vi "Cross Array Main.vi"() -> ()   [LabVIEW 2014]
uses:
  Slicer/LVslicer/Slice/TypeDefs/PowerSpeed.ctl
  Slicer/LVslicer/Slice/TypeDefs/PathSupreme.ctl
  Slicer/LVslicer/Slice/OverhangParam/PSup2SCAN/Sub/VelocityProfile.ctl
  Slicer/LVslicer/Slice/OverhangParam/PSup2SCAN/Sub/PathCut.ctl
  Slicer/LVslicer/Slice/OverhangParam/PSup2SCAN/Sub/Segment.ctl
  Slicer_11-28/LVslicer/Slice/TypeDefs/Point3D.ctl
  <vilib>/picture/3D Picture Control/Object/Create Object (name).vi
  <vilib>/picture/3D Picture Control/NI_3D Picture Control.lvlib
panel:
  in  "Layer Thickness":dbl
  in  "Path":path
  out "PathSupreams":T1[](array[typedef])
  in  "save":bool
  in  "Spacing":dbl
  in  "Plate \nDiameter":dbl
  out "Stoped":bool
  in  "HighPower":dbl=500.0
  in  "Display":T5={"Mode"=enum."Inherit Value", "PointSize"=1.0, "LineWidth"=1.0}
  out "3D Picture":refnum<vi>(3d-picture)
  out "PathSupreme":T1
  in  "stop":bool
  in  "Create Array":bool
  in  "Create Cross":bool
  in  "Beam Width":dbl
  in  "Cross X dimension\n(cross is square)":dbl
  in  "HatchPower":T6={"Power"=300.0, "Mark Speed"=400.0, "Jump Speed"=1000.0}
  # "* All dimensions are in mm's"
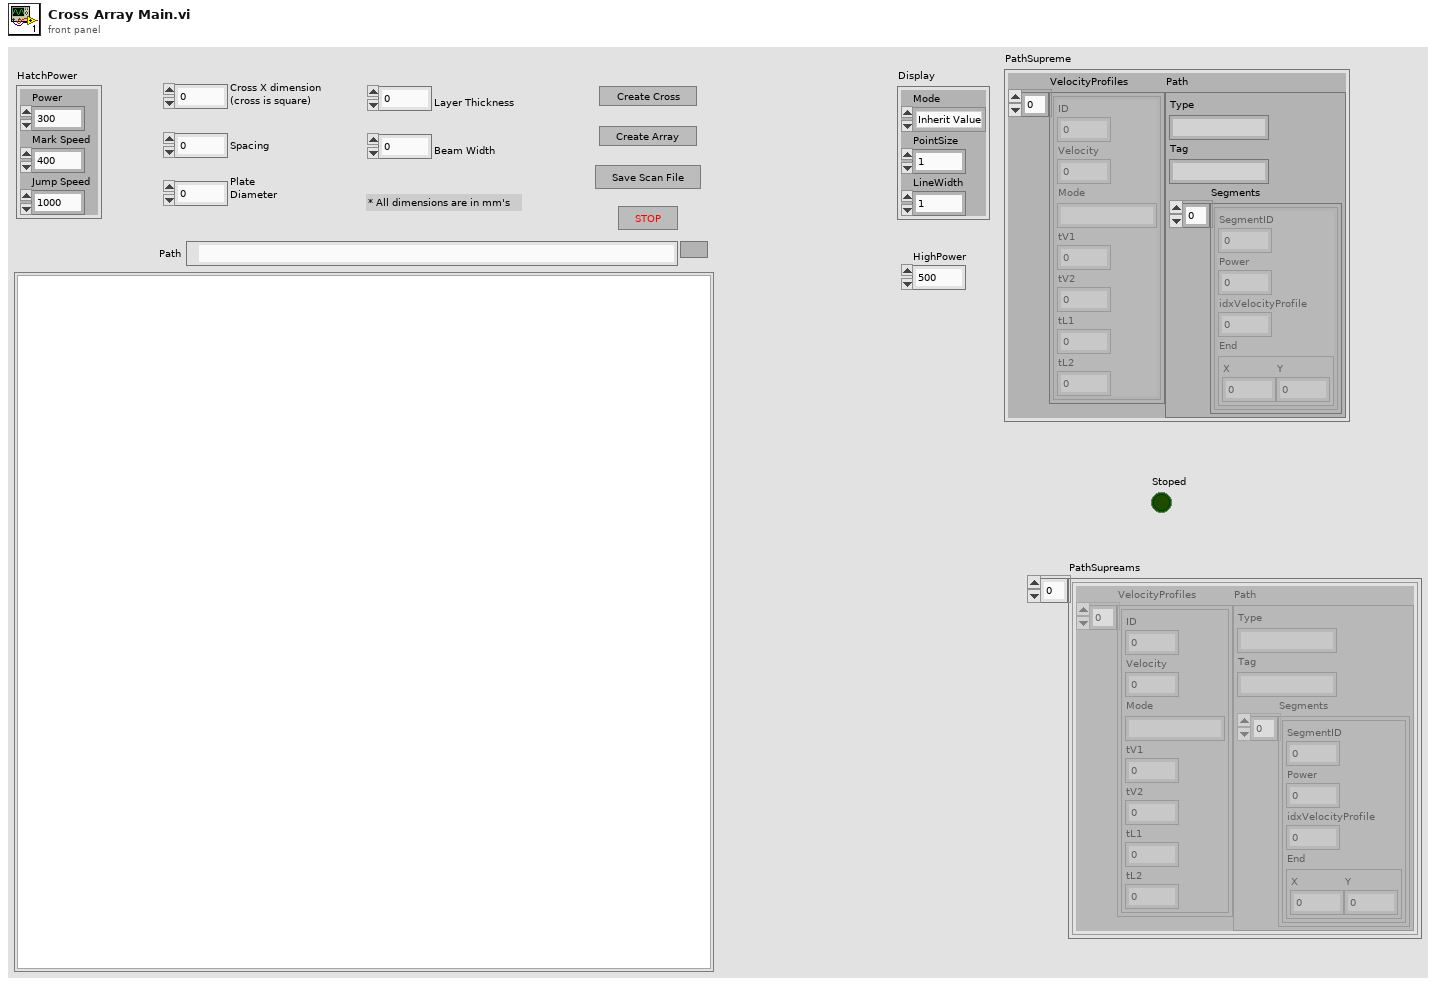
[diagram p1: front panel]
types:
  T1 = typedef "PathSupreme.ctl" = cluster{"VelocityProfiles":T2[], "Path":T3}
  T2 = typedef "VelocityProfile.ctl" = cluster{"ID":u32, "Velocity":dbl, "Mode":string, "tV1":u32, "tV2":u32, "tL1":u32, "tL2":u32}
  T3 = typedef "PathCut.ctl" = cluster{"Type":string, "Tag":string, "Segments":T4[]}
  T4 = typedef "Segment.ctl" = cluster{"SegmentID":u16, "Power":sgl, "idxVelocityProfile":u16, "End":cluster{"X":sgl, "Y":sgl}}
  T5 = cluster{"Mode":enum16{"Inherit Value", "Points", "Wireframe", "Polygons"}, "PointSize":sgl, "LineWidth":sgl}
  T6 = typedef "PowerSpeed.ctl" = cluster{"Power":dbl, "Mark Speed":dbl, "Jump Speed":dbl}
  T7 = typedef "Point3D.ctl" = cluster{"X":sgl, "Y":sgl, "Z":sgl}
  T8 = cluster{"Lines":cluster{"P0":T7, "P1":T7}[], "Colors":u32[]}
  T9 = enum16{"Idle", "Wait", "Create Cross", "Create Array", "Stop"}
  T10 = typedef "Point2DwSlope.ctl" = cluster{"X":sgl, "Y":sgl, "Slope":dbl}
  T11 = cluster{"VertexArray":T10[], "OnOffAr":enum16{"On", "Off"}[]}
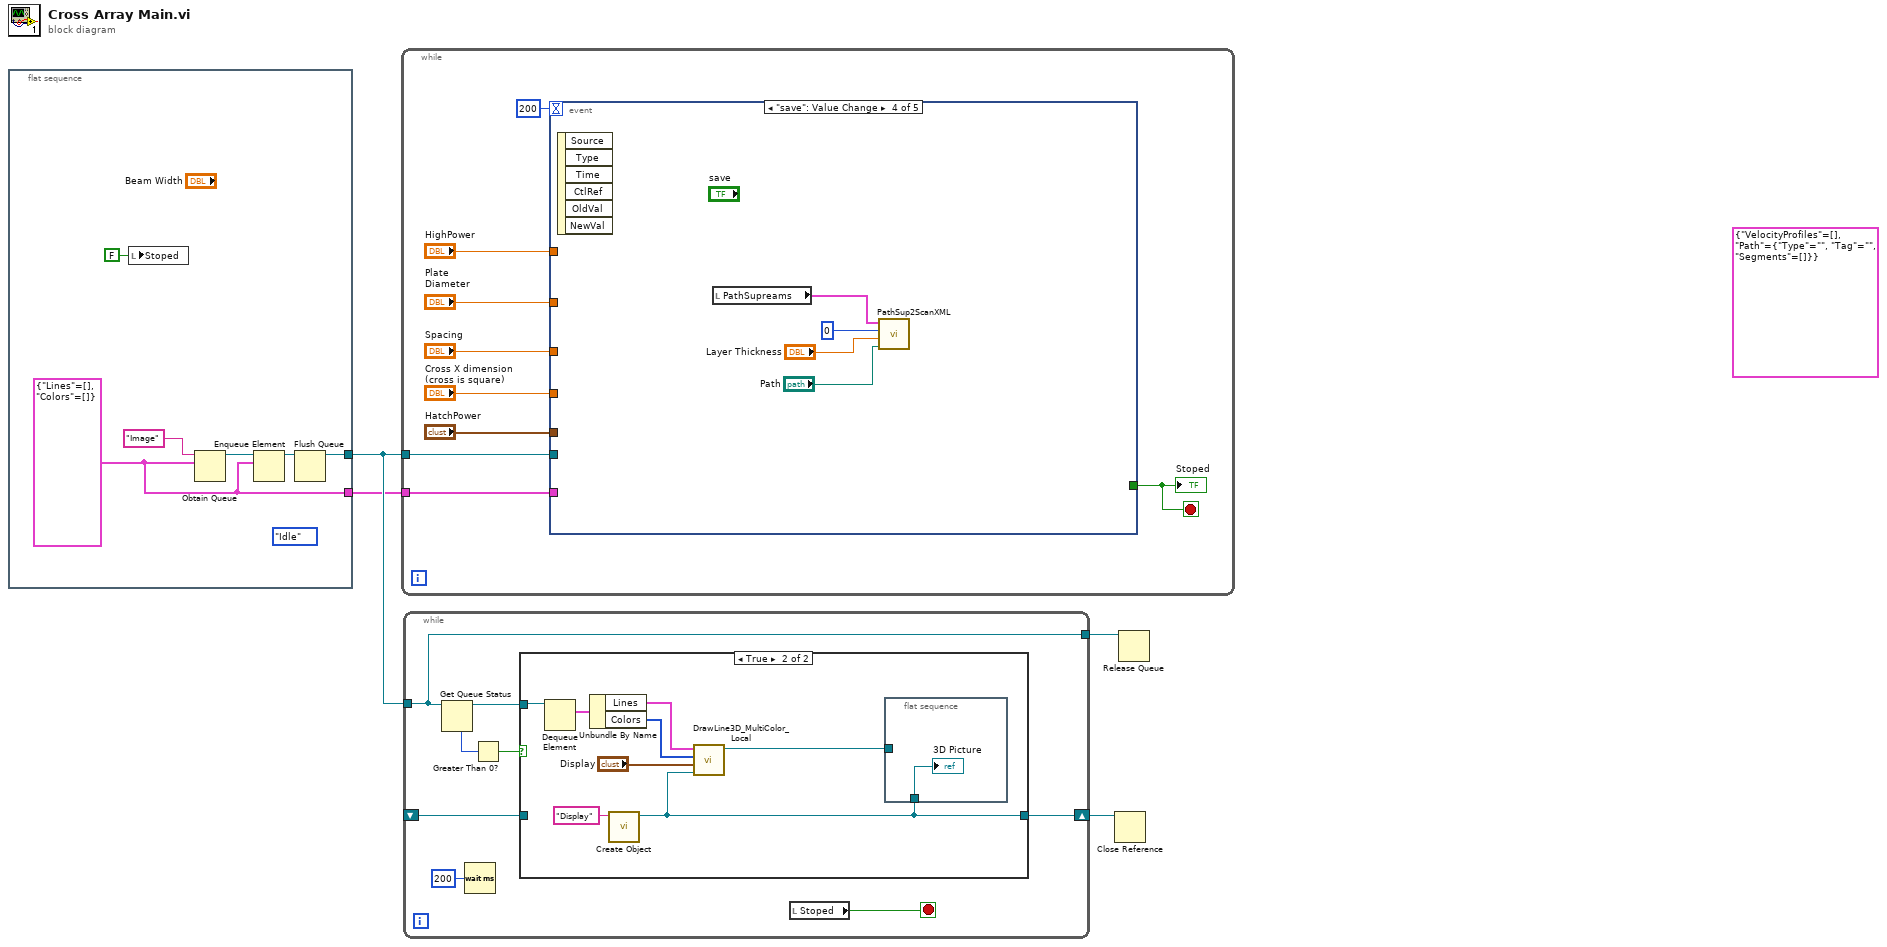
[diagram p0: block diagram]
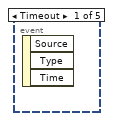
[diagram p2: hidden frame]
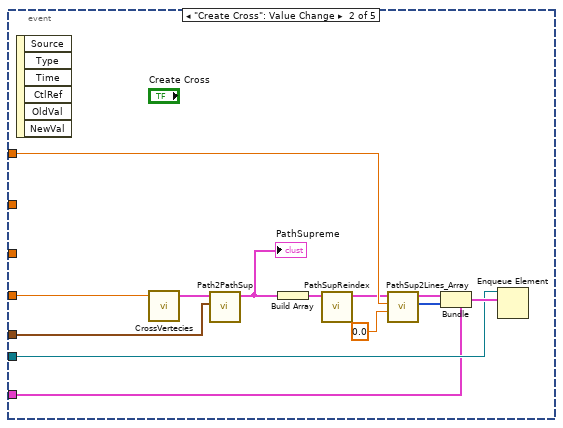
[diagram p3: hidden frame]
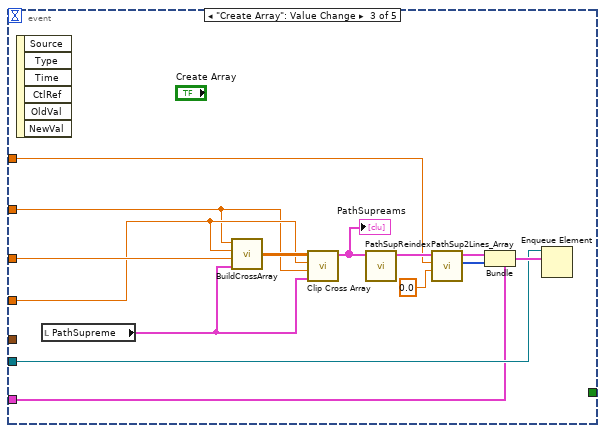
[diagram p4: hidden frame]
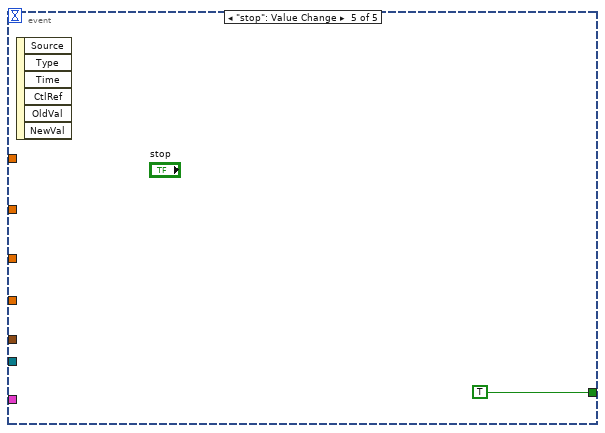
[diagram p5: hidden frame]
diagram:
  (unwired) T1 {"VelocityProfiles"=[], "Path"={"Type"="", "Tag"="", "Segments"=[]}} ("PathSupreme")
  n1 = flat-sequence {
    tunnel: [w7] -> w4
    tunnel: [w6] -> w3
    frame #0 {
      w6 = T8 {"Lines"=[], "Colors"=[]} ("output cluster")
      (unwired) T9."Idle" ("Action")
      n2 = local write "Stoped"(FALSE ("Stoped")) -> ()
      n3 = Obtain Queue(name (unnamed)="Image", element data type=w6) -> (queue out=w9:refnum<queue>)  [unwired: 3 in, 2 out]
      n4 = Enqueue Element(queue=w9, element=w6) -> (queue out=w8:refnum<queue>)  [unwired: 2 in, 2 out]
      n5 = Flush Queue(queue=w8) -> (queue out=w7:refnum<queue>)  [unwired: 1 in, 2 out]
    }
  }
  n6 = while {
    tunnel: w4 -> [w13]
    tunnel: w3 -> [w19]
    stop <- w18 stop-if-true
    n7 = event shown="[3] \"save\": Value Change" {
      selector: _ -> [_ _ _ _ _]
      dyn-events: _ -> [_ _ _ _ _]
      timeout: 200 -> [_ _ _ _ _]
      tunnel: "HighPower" -> [_ w31 w40 _ _]
      tunnel: w13 -> [_ w24 w39 _ _]
      tunnel: w19 -> [_ w23 w38 _ _]
      tunnel: [_ _ _ _ TRUE] -> w18
      tunnel: "Cross X dimension\n(cross is square)" -> [_ w21 w36 _ _]
      tunnel: "HatchPower" -> [_ w20 _ _ _]
      tunnel: "Plate \nDiameter" -> [_ _ w35 _ _]
      tunnel: "Spacing" -> [_ _ w46 _ _]
      event Timeout {
        n8 = event-data() -> ()  [unwired: 1 in, 3 out]
      }
      event "Create Cross": Value Change {
        n9 = event-data() -> ()  [unwired: 1 in, 6 out]
        n10 = call "CrossVertecies.vi"("Cross X dimension\n(cross is square)"=w21) -> ("Combined"=w32:T11)  [unwired: 4 in]
        n11 = call "Path2PathSup.vi"("PowerSpeed"=w20, "Combined"=w32) -> ("PathSupreme"=w22:T1)  [unwired: 9 in]
        "PathSupreme" <- w22
        n12 = Build Array(w22) -> (w28:T1[])
        n13 = call "PathSupReindex.vi"("PathSupremes"=w28) -> ("PathSupOut"=w29:T1[])  [unwired: 10 in]
        n14 = call "PathSup2Lines_Array.vi"("Z"=0.0, "HighPower"=w31, "PathSupIn"=w29) -> ("Colors"=w26:u32[], "Lines"=w27:cluster{"P0":T7, "P1":T7}[])  [unwired: 7 in]
        n15 = Bundle(cluster=w23, "Lines"=w27, "Colors"=w26) -> (w25:T8)
        n16 = Enqueue Element(queue=w24, element=w25) -> ()  [unwired: 2 in, 3 out]
      }
      event "Create Array": Value Change {
        n17 = event-data() -> ()  [unwired: 1 in, 6 out]
        n18 = local read "PathSupreme"() -> (w34:T1)
        n19 = call "BuildCrossArray.vi"("Plate \nDiameter (mm)"=w35, "Cross X dimension\n(cross is square)"=w36, "Desired\nSpacing(mm)"=w46, "PathSupreme"=w34) -> ("Array 2"=w37:dbl[][])  [unwired: 3 in, 1 out]
        n20 = call "Clip Cross Array.vi"("PathSupreme"=w34, "Plate \nDiameter (mm)"=w35, "Cross X dimension\n(cross is square)"=w36, "Origion Array"=w37) -> ("PathSupreams"=w33:T1[])  [unwired: 4 in]
        "PathSupreams" <- w33
        n21 = call "PathSupReindex.vi"("PathSupremes"=w33) -> ("PathSupOut"=w44:T1[])  [unwired: 10 in]
        n22 = call "PathSup2Lines_Array.vi"("Z"=0.0, "HighPower"=w40, "PathSupIn"=w44) -> ("Colors"=w42:u32[], "Lines"=w43:cluster{"P0":T7, "P1":T7}[])  [unwired: 7 in]
        n23 = Bundle(cluster=w38, "Lines"=w43, "Colors"=w42) -> (w41:T8)
        n24 = Enqueue Element(queue=w39, element=w41) -> ()  [unwired: 2 in, 3 out]
      }
      event "save": Value Change {
        n25 = event-data() -> ()  [unwired: 1 in, 6 out]
        n26 = local read "PathSupreams"() -> (w50:T1[])
        n27 = call "PathSup2ScanXML.vi"("PathSupremes"=w50, "layer"=u32 0, "Thickness"="Layer Thickness", "Path"="Path") -> ()  [unwired: 2 in, 1 out]
      }
      event "stop": Value Change {
        n28 = event-data() -> ()  [unwired: 1 in, 6 out]
      }
    }
    "Stoped" <- w18
  }
  n29 = while {
    tunnel: w4 -> [w55]
    tunnel: [w55] -> w1
    shift-right: [w53] -> w2
    shift-left: _ -> [w52]
    stop <- w54 stop-if-true
    n30 = Get Queue Status(queue=w55) -> (queue out=w58:refnum<queue>, # elements in queue=w57:i32)  [unwired: 2 in, 6 out]
    n31 = Wait (ms)(milliseconds to wait=u32 200) -> ()  [unwired: 1 out]
    n32 = Greater Than 0?(x=w57) -> (x > 0?=w56:bool)
    n33 = case shown="True" w56 {
      tunnel: w58 -> [_ w67]
      tunnel: [w60 w61] -> w53
      tunnel: w52 -> [w60 _]
      frame False {
      }
      frame True {
        n34 = Dequeue Element(queue=w67) -> (element=w66:T8)  [unwired: 2 in, 3 out]
        n35 = Unbundle By Name(w66) -> ("Lines"=w65:cluster{"P0":T7, "P1":T7}[], "Colors"=w64:u32[])
        n36 = call-poly <vilib>:"Create Object.vi"("Name"="Display") -> ("Scene:New Object"=w61:refnum<vi>)  [unwired: 9 in, 1 out]
        n37 = call "DrawLine3D_MultiColor_Local.vi"("Scene Object In"=w61, "Display"="Display", "Colors"=w64, "Lines"=w65) -> ("Scene Object Out"=w62:refnum<vi>)  [unwired: 7 in]
        n38 = flat-sequence {
          tunnel: w61 -> [w69]
          tunnel: w62 -> [_]
          frame #0 {
            "3D Picture" <- w69
          }
        }
      }
    }
    n39 = local read "Stoped"() -> (w54:bool)
  }
  n40 = Close Reference(reference=w2) -> ()  [unwired: 1 in, 1 out]
  n41 = Release Queue(queue=w1) -> ()  [unwired: 2 in, 3 out]
